vi "行删除.vi"(8 "error in (no error)":errorcluster caption="错误输入（无错误）", 11 "程序响应 输入":refnum<class "程序响应.lvclass">) -> (0 "error out":errorcluster caption="错误输出", 3 "程序响应 输出":refnum<class "程序响应.lvclass">)   [LabVIEW 2020, in "程序响应.lvlib" / "程序响应.lvclass"]
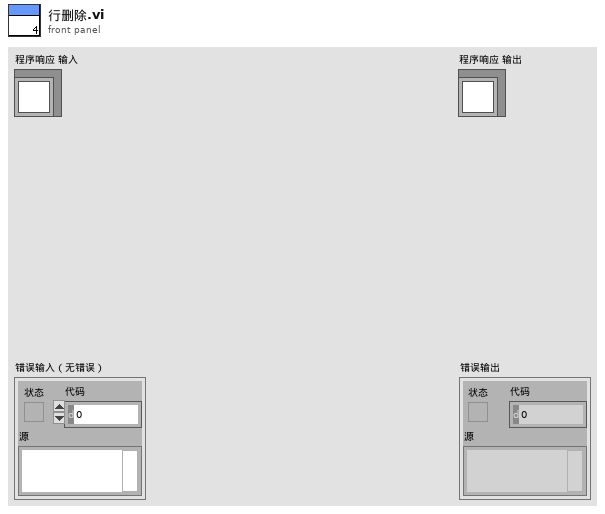
[diagram p1: front panel]
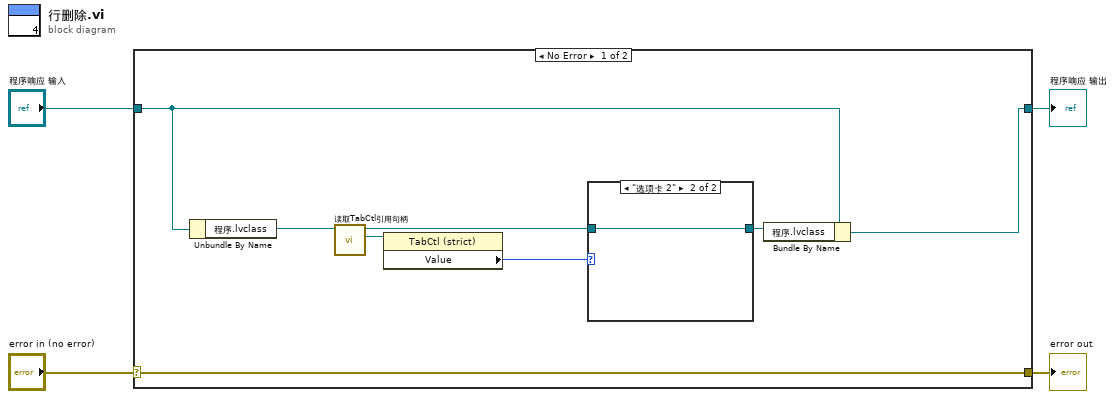
[diagram p0: block diagram]
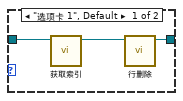
[diagram p2: hidden frame]
diagram:
  n1 = case shown="No Error" "error in (no error)" {
    selector: "error in (no error)" -> [w12 w18]
    tunnel: [w12 w18] -> w3
    tunnel: [w9 w17] -> w1
    tunnel: "程序响应 输入" -> [w10 w17]
    frame No Error {
      n2 = Unbundle By Name(w10) -> ("程序.lvclass"=w7:refnum<class "程序.lvclass">)
      n3 = call-dynamic "读取TabCtl引用句柄.vi"("程序输入"=w7) -> ("TabCtl引用句柄"=w8:refnum<vi>, "程序输出"=w6:refnum<class "程序.lvclass">)  [unwired: 8 in, 1 out]
      n4 = property class="TabCtl (strict)"(reference=w8) -> ("Value"=w5:enum32{"选项卡 1", "选项卡 2"})  [unwired: 1 in, 2 out]
      n5 = case shown="\"选项卡 2\"" w5 {
        tunnel: [w14 w16] -> w11
        tunnel: w6 -> [w13 w16]
        frame "选项卡 1", Default {
          n6 = call-dynamic "获取索引.vi"("程序 输入"=w13) -> ("程序 输出"=w15:refnum<class "程序.lvclass">)  [unwired: 9 in, 1 out]
          n7 = call-dynamic "行删除.vi"("程序 输入"=w15) -> ("程序 输出"=w14:refnum<class "程序.lvclass">)  [unwired: 9 in, 1 out]
        }
        frame "选项卡 2" {
        }
      }
      n8 = Bundle By Name(cluster=w10, "程序.lvclass"=w11) -> (w9:refnum<class "程序响应.lvclass">)
    }
    frame Error {
    }
  }
  "error out" <- w3
  "程序响应 输出" <- w1
